vi "单选按钮（允许不选）.vi"() -> ()   [LabVIEW 2012]
panel:
  out "Port":u8 format="%.0x"
  out "Line":bool[](array[boolean])
  in  "DO":T1(radio)=enum."单选选项1"
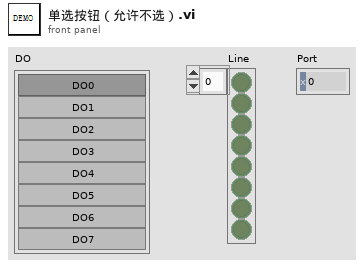
[diagram p1: front panel]
types:
  T1 = enum32{"未选择", "单选选项1", "单选选项1 2", "单选选项1 3", "单选选项1 4", "单选选项1 5", "单选选项1 6", "单选选项1 7", "单选选项1 8"}
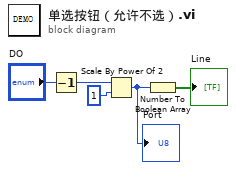
[diagram p0: block diagram]
diagram:
  n1 = Decrement(x="DO") -> (x-1=w2:T1)
  n2 = Scale By Power Of 2(n=w2, x=u8 1) -> (x*2^n=w3:u8)
  "Port" <- w3
  n3 = Number To Boolean Array(number=w3) -> (Boolean array=→"Line":bool[])
